vi "WAV_Chunk.vi"(9 "data string":string, 11 "string":string) -> (1 "String out":string)   [LabVIEW 2022 SP3]
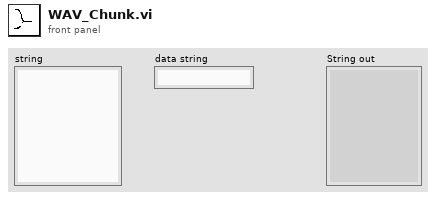
[diagram p1: front panel]
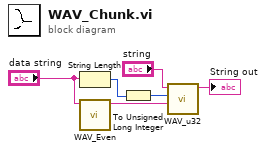
[diagram p0: block diagram]
diagram:
  n1 = String Length(string="data string") -> (length=w3:i32)
  n2 = call "WAV_Even.vi"("string in"="data string") -> ("string out"=w4:string)  [unwired: 10 in]
  n3 = To Unsigned Long Integer(number=w3) -> (unsigned 32bit integer=w6:u32)
  n4 = call "WAV_u32.vi"("data string"=w4, "u32"=w6, "String in"="string") -> ("String out"=→"String out":string)  [unwired: 8 in]
